vi "Write ConfigurationData.vi"(8 "error in (no error)":errorcluster, 10 "ConfigurationData":string, 11 "ENET_BS120x in":refnum<class "ENET_BS120x.lvclass">) -> (0 "error out":errorcluster, 3 "ENET_BS120x out":refnum<class "ENET_BS120x.lvclass">)   [LabVIEW 2021, in "BS120x Driver.lvlib" / "ENET_BS120x.lvclass"]
uses:
  ENET_BS120x.lvclass
  ENET_BS120x.lvclass/ENET_BS120x.ctl
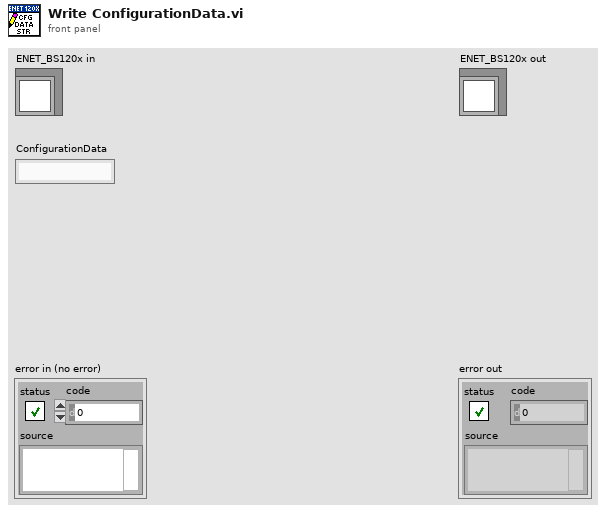
[diagram p1: front panel]
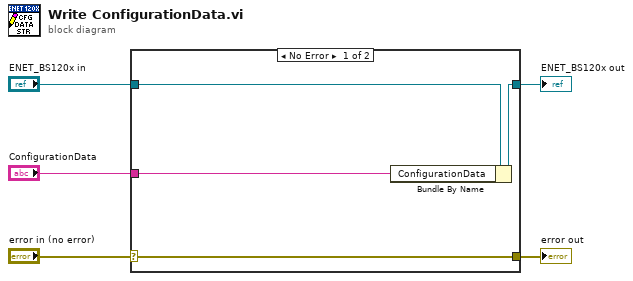
[diagram p0: block diagram]
diagram:
  n1 = case shown="No Error" "error in (no error)" {
    selector: "error in (no error)" -> [w9 w10]
    tunnel: [w9 w10] -> w4
    tunnel: [w7 w11] -> w2
    tunnel: "ENET_BS120x in" -> [w8 w11]
    tunnel: "ConfigurationData" -> [w6 _]
    frame No Error {
      n2 = Bundle By Name(cluster=w8, "ConfigurationData"=w6) -> (w7:refnum<class "ENET_BS120x.lvclass">)
    }
    frame Error {
    }
  }
  "error out" <- w4
  "ENET_BS120x out" <- w2
